vi "From HW.vi"(5 "Plot window":string) -> (0 "Y name":string, 1 "Y # signal":string, 2 "Ready?":bool)   [LabVIEW 2022 SP3]
panel:
  out "Clone Name":string
  in  "Close windows":bool
  in  "Y data":string(combo)
  in  "Add":bool
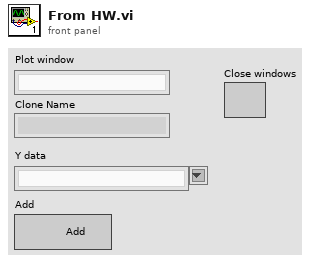
[diagram p1: front panel]
types:
  T1 = enum32{"Invalid", "Standard", "Closed", "Hidden", "Minimized", "Maximized"}
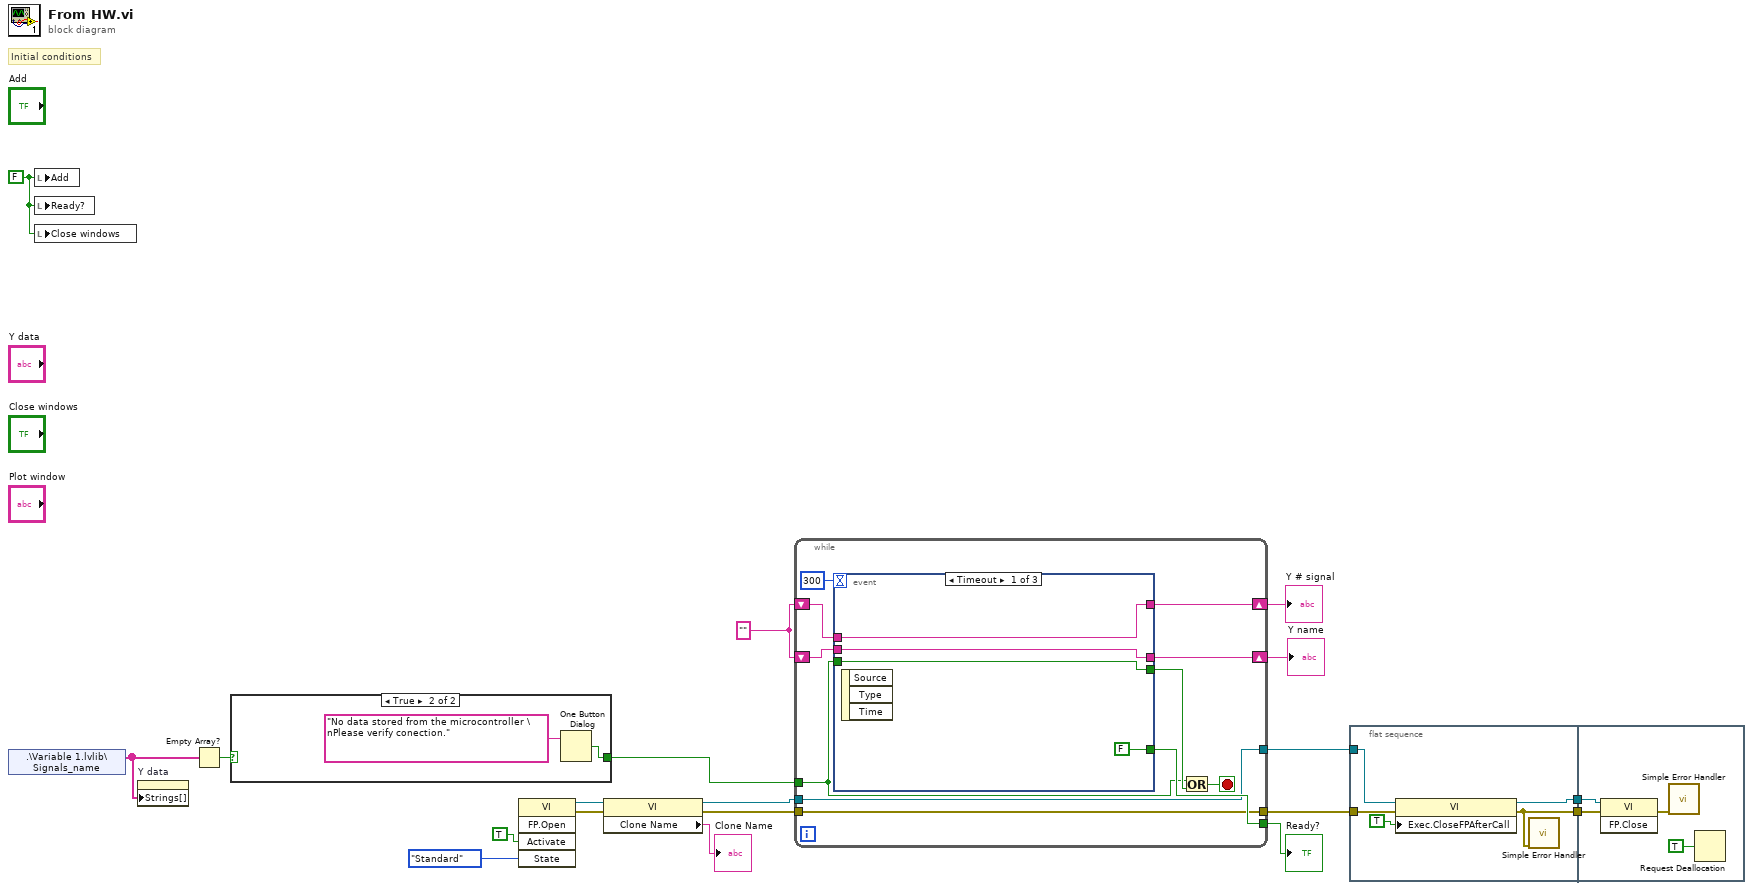
[diagram p0: block diagram]
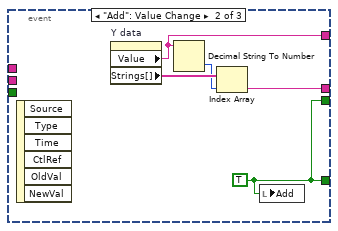
[diagram p3: hidden frame]
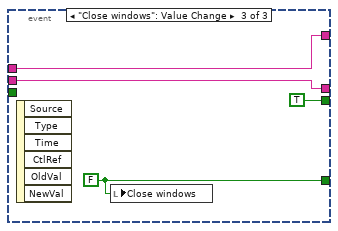
[diagram p4: hidden frame]
diagram:
  w2 = "" ("Value")
  w8 = FALSE
  # "Initial conditions"
  n1 = shared-variable ".\\Variable 1.lvlib\\Signals_name"() -> (w7:string[])  [unwired: 1 in, 1 out]
  n2 = local write "Add"(w8) -> ()
  n3 = local write "Ready?"(w8) -> ()
  n4 = local write "Close windows"(w8) -> ()
  n5 = property on="Y data" class="CmbBox"("Strings[]"=w7) -> ()  [unwired: 2 in, 2 out]
  n6 = Empty Array?(array=w7) -> (empty?=w6:bool)
  n7 = case shown="True" w6 {
    selector: w6 -> [w20 _]
    tunnel: [w20 w21] -> w5
    frame False {
    }
    frame True {
      n8 = One Button Dialog(message="No data stored from the microcontroller \nPlease verify conection.") -> (true=w21:bool)  [unwired: 1 in]
    }
  }
  n9 = invoke on="Invoke Node" class="VI" method="FP.Open"("Activate"=TRUE ("Activate?"), "State"=T1."Standard") -> (reference out=w15:refnum<vi>, error out=w16:errorcluster)  [unwired: 3 in, 3 out]
  n10 = property on="Property Node" class="VI"(reference=w15, error in=w16) -> (reference out=w14:refnum<vi>, error out=w17:errorcluster, "Clone Name"=→"Clone Name":string)
  n11 = while {
    tunnel: [w33] -> w19
    tunnel: w17 -> [w32]
    tunnel: w14 -> [w27]
    tunnel: [w27] -> w12
    tunnel: [w32] -> w11
    tunnel: w5 -> [w25]
    shift-right: [w31] -> w3
    shift-left: w2 -> [w30]
    shift-right: [w29] -> w4
    shift-left: w2 -> [w28]
    stop <- w24 stop-if-true
    n12 = event shown="[0] Timeout" {
      selector: _ -> [_ _ _]
      dyn-events: _ -> [_ _ _]
      timeout: 300 -> [_ _ _]
      tunnel: [w35 w38 TRUE] -> w26
      tunnel: [FALSE w38 w45] -> w33
      tunnel: [w37 w42 w44] -> w31
      tunnel: w30 -> [w37 _ w44]
      tunnel: [w36 w39 w43] -> w29
      tunnel: w28 -> [w36 _ w43]
      tunnel: w25 -> [w35 _ _]
      event Timeout {
        n13 = event-data() -> ()  [unwired: 1 in, 3 out]
      }
      event "Add": Value Change {
        w38 = TRUE
        n14 = event-data() -> ()  [unwired: 1 in, 6 out]
        n15 = property on="Y data" class="CmbBox"() -> ("Value"=w42:string, "Strings[]"=w41:string[])  [unwired: 2 in, 2 out]
        n16 = Decimal String To Number(string=w42) -> (number=w40:i32)  [unwired: 2 in, 1 out]
        n17 = Index Array(array=w41, index=w40) -> (element=w39:string)
        n18 = local write "Add"(w38) -> ()
      }
      event "Close windows": Value Change {
        w45 = FALSE
        n19 = event-data() -> ()  [unwired: 1 in, 6 out]
        n20 = local write "Close windows"(w45) -> ()
      }
    }
    n21 = Or(x=w25, y=w26) -> (x .or. y?=w24:bool)
  }
  "Ready?" <- w19
  "Y name" <- w4
  "Y # signal" <- w3
  n22 = flat-sequence {
    tunnel: w12 -> [w51]
    tunnel: w11 -> [w50]
    tunnel: [w48] -> w10
    tunnel: [w47] -> w9
    tunnel: w10 -> [w54]
    tunnel: w9 -> [w53]
    frame #0 {
      n23 = property class="VI"(reference=w51, error in=w50, "Exec.CloseFPAfterCall"=TRUE ("Activate?")) -> (reference out=w48:refnum<vi>, error out=w47:errorcluster)
      n24 = call <vilib>:"Simple Error Handler.vi"("error in (no error)"=w47) -> ()  [unwired: 4 in, 5 out]
    }
    frame #1 {
      n25 = invoke class="VI" method="FP.Close"(reference=w54, error in=w53) -> (error out=w55:errorcluster)  [unwired: 1 in, 2 out]
      n26 = call <vilib>:"Simple Error Handler.vi"("error in (no error)"=w55) -> ()  [unwired: 4 in, 5 out]
      n27 = Request Deallocation(TRUE ("flag")) -> ()
    }
  }
